vi "Set_Ao.vi"(0 "reference in":refnum<class "Sig_AO.lvclass">, 5 "AO":dbl, 11 "error in (no error)":errorcluster) -> (4 "reference out":refnum<class "Sig_AO.lvclass">, 15 "error out":errorcluster)   [LabVIEW 2019, in "Sig_AO.lvclass"]
uses:
  Sig_AO.lvclass
  D:/H4000/src/Proccess_class/Proccess.lvclass
  Sig_AO.lvclass/Sig_AO.ctl
  Proccess_class/Proccess.lvclass/Proccess.ctl
  Logger_class/Logger.lvclass/Logger.ctl
  Logger_class/Enqueue Signal.vi
  Proccess_class/Read TagName.vi
  Proccess_class/Read Logger.vi
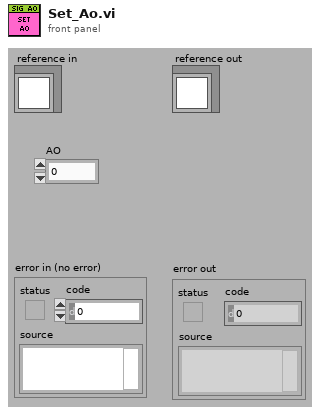
[diagram p1: front panel]
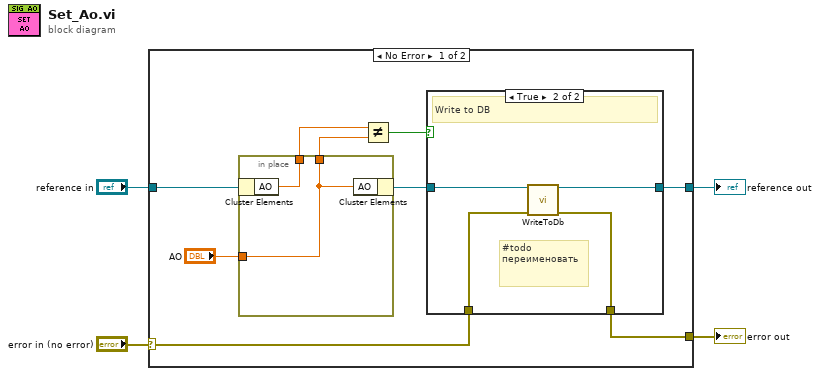
[diagram p0: block diagram]
diagram:
  n1 = case shown="No Error" "error in (no error)" {
    selector: "error in (no error)" -> [w13 w23]
    tunnel: [w8 w23] -> w3
    tunnel: [w9 w22] -> w1
    tunnel: "reference in" -> [w11 w22]
    frame No Error {
      n2 = in-place {
        in-place-border: "AO" -> [w20]
        in-place-border: [w21] -> w6
        in-place-border: [w20] -> w5
        n3 = in-place-cluster #1(w11) -> ("AO"=w21:dbl)
        n4 = in-place-cluster #1("AO"=w20) -> (w10:refnum<class "Sig_AO.lvclass">)
      }
      n5 = Not Equal?(x=w6, y=w5) -> (x != y?=w12:bool)
      n6 = case shown="True" w12 {
        tunnel: w10 -> [w15 w19]
        tunnel: [w15 w18] -> w9
        tunnel: [w14 w16] -> w8
        tunnel: w13 -> [w14 w17]
        frame False {
        }
        frame True {
          # "#todo\nпереименовать"
          # "Write to DB"
          n7 = call "WriteToDb.vi"("reference in"=w19, "error in (no error)"=w17) -> ("reference out"=w18:refnum<class "Sig_AO.lvclass">, "error out"=w16:errorcluster)  [unwired: 12 in]
        }
      }
    }
    frame Error {
    }
  }
  "error out" <- w3
  "reference out" <- w1
